vi "CAN_enable_MAGIC.vi"(3 "error in (no error)":errorcluster, 4 "Current":i32(slide) scale=-1000.0..1000.0, 5 "sbCANopenBaseClass in":refnum<class "sbCANopenBaseClass.lvclass">) -> (0 "error out":errorcluster, 2 "CANopen Session Out":refnum<class "sbCANopenBaseClass.lvclass">)   [LabVIEW 2024]
uses:
  <vilib>/addons/Maxon Motor/EPOS2 CANopen/CANopen/sbCANopenBaseClass.lvclass
  <vilib>/addons/Maxon Motor/EPOS2 CANopen/EPOS2 Support Files/Typedefs/EPOS2 Control Word PVM.ctl
  <vilib>/addons/Maxon Motor/EPOS2 CANopen/EPOS2 Support Files/Polymorphic SubVIs/Write PDO/EPOS2 Current Mode Write.vi
  <vilib>/addons/Maxon Motor/EPOS2 CANopen/EPOS2 Library.lvlib
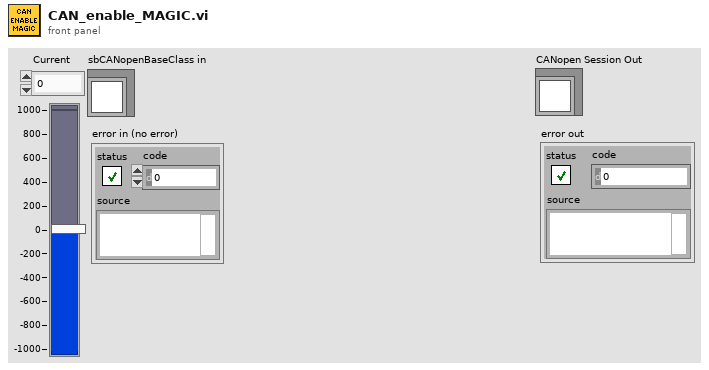
[diagram p1: front panel]
types:
  T1 = typedef "EPOS2 Library.lvlib/EPOS2 Control Word PVM.ctl" = cluster{"Switch On":bool, "Enable Voltage":bool, "Quick Stop":bool, "Enable Operation":bool, "Reserved 0":bool, "Reserved 1":bool, "Reserved 2":bool, "Fault Reset":bool, "Halt":bool}
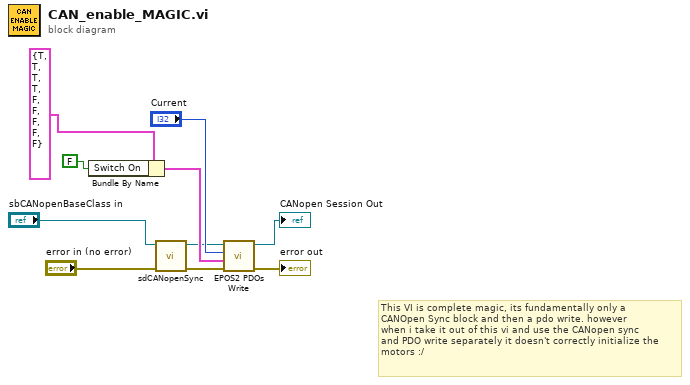
[diagram p0: block diagram]
diagram:
  # "This VI is complete magic, its fundamentally only a \nCANOpen Sync block and then a pdo write. however \nwhen i take it out of this vi and use the CANopen sync \nand PDO write separately it doesn't correctly initialize the\nmotors :/"
  n1 = Bundle By Name(cluster=T1 {"Switch On"=TRUE, "Enable Voltage"=TRUE, "Quick Stop"=TRUE, "Enable Operation"=TRUE, "Reserved 0"=FALSE, "Reserved 1"=FALSE, "Reserved 2"=FALSE, "Fault Reset"=FALSE, "Halt"=FALSE} ("Control Word"), "Switch On"=FALSE) -> (w8:T1)
  n2 = call-dynamic "sdCANopenSync.vi"("error in (no error)"="error in (no error)", "sbCANopenBaseClass in"="sbCANopenBaseClass in") -> ("error out"=w1:errorcluster, "sbCANopenBaseClass out"=w2:refnum<class "sbCANopenBaseClass.lvclass">)  [unwired: 8 in]
  n3 = call-poly <vilib>:"EPOS2 PDOs Write.vi"("error in"=w1, "Control Word"=w8, "Current"="Current", "CANopen Session In"=w2) -> ("error out"=→"error out":errorcluster, "CANopen Session Out"=→"CANopen Session Out":refnum<class "sbCANopenBaseClass.lvclass">)  [unwired: 6 in]
